vi "Save Data.vi"(8 "error in (no error)":errorcluster, 11 "RP I-V Driver in":refnum<class "RP I-V Driver.lvclass">) -> (0 "error out":errorcluster, 1 "Finished":bool, 2 "Current read position":i32, 3 "RP I-V Driver out":refnum<class "RP I-V Driver.lvclass">)   [LabVIEW 2020, in "RP I-V Driver.lvclass"]
uses:
  Instruments/Pulse Driver/Pulse Driver.lvclass/Pulse Driver.ctl
  Instruments/Pulse Driver/Read Current read position.vi
  RP I-V Driver.lvclass
  RP I-V Driver.lvclass/RP I-V Driver.ctl
  RP Instrument/RP Instrument.lvclass
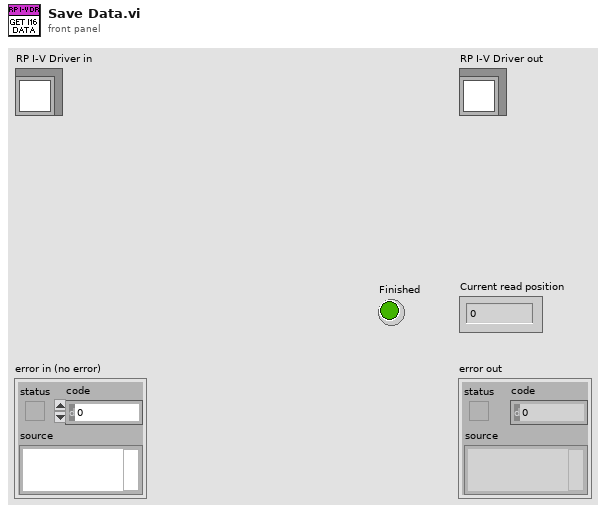
[diagram p1: front panel]
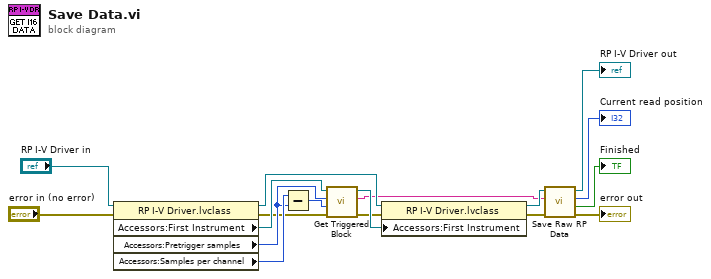
[diagram p0: block diagram]
diagram:
  n1 = property class="RP I-V Driver.lvclass"(reference="RP I-V Driver in", error in="error in (no error)") -> (reference out=w17:refnum<class "RP I-V Driver.lvclass">, error out=w12:errorcluster, "Accessors:First Instrument"=w16:refnum<class "RP Instrument.lvclass">, "Accessors:Pretrigger samples"=w14:u32, "Accessors:Samples per channel"=w15:i32)
  n2 = Subtract(x=w15, y=w14) -> (x-y=w13:u32)
  n3 = call-dynamic "Get Triggered Block.vi"("error in (no error)"=w12, "Post-trigger points"=w13, "Pre-trigger points"=w14, "RP Instrument in"=w16) -> ("error out"=w10:errorcluster, "Data out"=w7:string, "RP Instrument out"=w11:refnum<class "RP Instrument.lvclass">)  [unwired: 5 in]
  n4 = property class="RP I-V Driver.lvclass"(reference=w17, error in=w10, "Accessors:First Instrument"=w11) -> (reference out=w9:refnum<class "RP I-V Driver.lvclass">, error out=w8:errorcluster)
  n5 = call-dynamic "Save Raw RP Data.vi"("error in (no error)"=w8, "Raw data"=w7, "RP I-V Driver in"=w9) -> ("error out"=→"error out":errorcluster, "Finished"=→"Finished":bool, "Current read position"=→"Current read position":i32, "RP I-V Driver out"=→"RP I-V Driver out":refnum<class "RP I-V Driver.lvclass">)  [unwired: 5 in]
